vi "temp con.vi"() -> ()   [LabVIEW 2018]
panel:
  out "MANUAL\nOVER RIDE":bool
  in  "stop":bool
  out "temp":dbl(slide) scale=0.0..100.0
  out "T > SP":bool
  out "T = SP":bool
  out "T < SP":bool
  out "Operational\nMode":string
  in  "MAN/AUTO":bool
  out "Deg C":dbl
  in  "Manual\nOverRide":bool
  out "Heater":bool
  in  "Deg C":dbl
  out "Set-Point":dbl(slide) scale=0.0..100.0
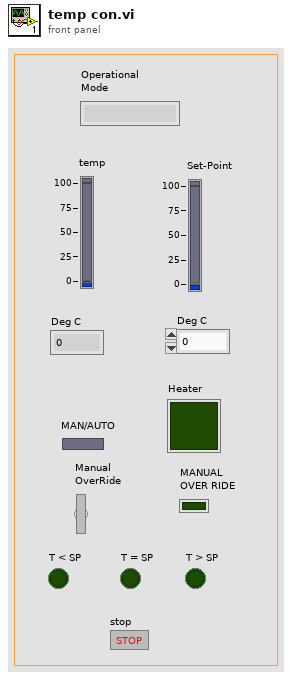
[diagram p1: front panel]
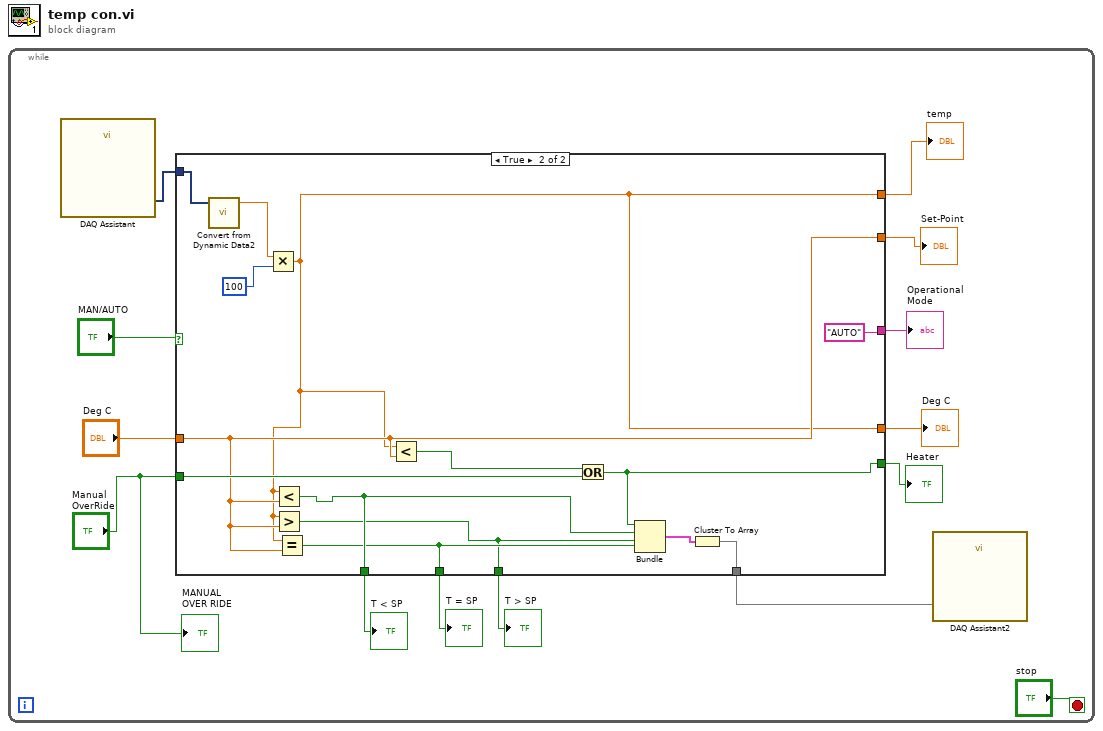
[diagram p0: block diagram]
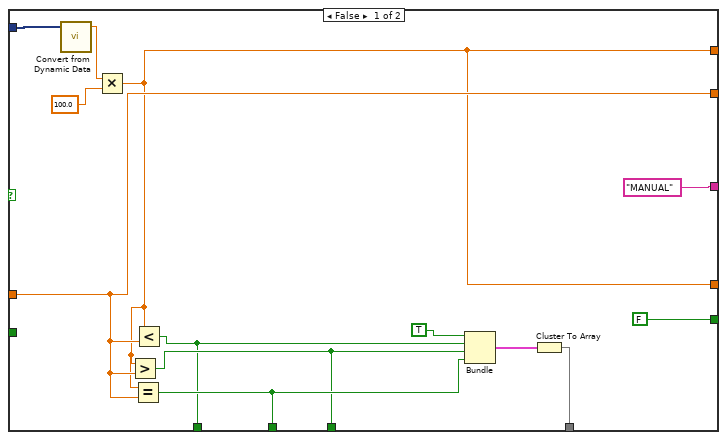
[diagram p2: hidden frame]
diagram:
  n1 = while {
    stop <- "stop" stop-if-true
    n2 = call "DAQ Assistant"() -> ("data"=w10:dynamicdata)  [unwired: 17 in, 2 out]
    n3 = case shown="True" "MAN/AUTO" {
      tunnel: ["MANUAL" "AUTO"] -> w13
      tunnel: [w16 w29] -> w12
      tunnel: "Deg C" -> [w16 w29]
      tunnel: "Manual\nOverRide" -> [_ w39]
      tunnel: w10 -> [w26 w38]
      tunnel: [w15 w28] -> w9
      tunnel: [w15 w28] -> w8
      tunnel: [FALSE w31] -> w7
      tunnel: [w18 w36] -> w4
      tunnel: [w22 w35] -> w6
      tunnel: [w21 w34] -> w5
      tunnel: [w19 w33] -> w3
      frame False {
        n4 = call "Convert from Dynamic Data"("Dynamic Data Type"=w26) -> ("Scalar"=w25:dbl)  [unwired: 3 in]
        n5 = Multiply(x=w25, y=100.0) -> (x*y=w15:dbl)
        n6 = Greater?(x=w15, y=w16) -> (0:w21:bool)
        n7 = Equal?(x=w15, y=w16) -> (x = y?=w22:bool)
        n8 = Less?(x=w15, y=w16) -> (x < y?=w18:bool)
        n9 = Bundle(TRUE, w18, w21, w22) -> (w20:cluster{bool, bool, bool, bool})  [unwired: 1 in]
        n10 = Cluster To Array(cluster=w20) -> (array=w19:bool[])
      }
      frame True {
        n11 = call "Convert from Dynamic Data2"("Dynamic Data Type"=w38) -> ("Scalar"=w37:dbl)  [unwired: 3 in]
        n12 = Multiply(x=w37, y=100) -> (x*y=w28:dbl)
        n13 = Less?(x=w28, y=w29) -> (x < y?=w36:bool)
        n14 = Greater?(x=w28, y=w29) -> (0:w34:bool)
        n15 = Equal?(x=w28, y=w29) -> (x = y?=w35:bool)
        n16 = Less?(x=w28, y=w29) -> (x < y?=w30:bool)
        n17 = Or(x=w30, y=w39) -> (x .or. y?=w31:bool)
        n18 = Bundle(w31, w36, w34, w35) -> (w32:cluster{bool, bool, bool, bool})  [unwired: 1 in]
        n19 = Cluster To Array(cluster=w32) -> (array=w33:bool[])
      }
    }
    "Set-Point" <- w12
    "Heater" <- w7
    "Deg C" <- w8
    "Operational\nMode" <- w13
    "T < SP" <- w4
    "T = SP" <- w6
    "T > SP" <- w5
    "temp" <- w9
    n20 = call "DAQ Assistant2"("data"=w3) -> ()  [unwired: 17 in, 2 out]
    "MANUAL\nOVER RIDE" <- "Manual\nOverRide"
  }
